vi "Hex Encode String.vi"(11 "String":string) -> (3 "Hex Encoded String":string)   [LabVIEW 2020, in "Crypto.lvlib"]
uses:
  Crypto.lvlib
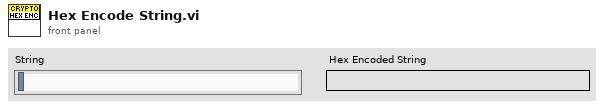
[diagram p1: front panel]
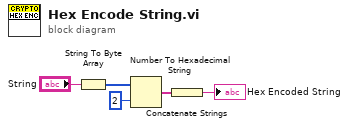
[diagram p0: block diagram]
diagram:
  n1 = String To Byte Array(string="String") -> (unsigned byte array=w4:u8[])
  n2 = Number To Hexadecimal String(1:i16 2 ("width (-)"), 2:w4) -> (0:w2:string[])
  n3 = Concatenate Strings(w2) -> (→"Hex Encoded String":string)
